vi "最大值比较器（I32).vi"(10 "reset":bool, 11 "Input":i32) -> (3 "Max":i32)   [LabVIEW 2012]
doc: "功能：\n\n根据输入的数值，连续比较输入的最大值。\n\n基本算法：\n\n利用LV2全局变量（反馈节点）存储上一次输入值，和本次输入值比较，返回最大值。\n\nCSXCS_366创建"
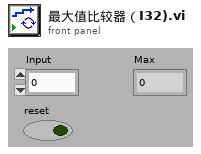
[diagram p1: front panel]
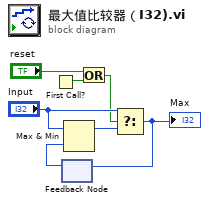
[diagram p0: block diagram]
diagram:
  n1 = First Call?() -> (First Call?: T/F=w3:bool)
  n2 = feedback #1() -> (w7:i32)  [unwired: 1 in]
  n3 = Max & Min(x="Input", y=w7) -> (max(x,y)=w1:i32)  [unwired: 1 out]
  n4 = Or(x="reset", y=w3) -> (x .or. y?=w2:bool)
  n5 = Select(t="Input", s=w2, f=w1) -> (s? t:f=w5:i32)
  "Max" <- w5
  n6 = feedback-in #1(w5) -> ()
